vi "Day 2.vi"() -> ()   [LabVIEW 2020]
uses:
  Direction_ENUM.ctl
  a7b40cfa-35c7-42bc-aad7-62f11c57efb3.vi
  <vilib>/Utility/file.llb/Read Delimited Spreadsheet (string).vi
  dc0bc9a9-6357-48e5-90de-08fc84681665.vi
panel:
  out "Position":i32
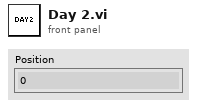
[diagram p1: front panel]
types:
  T1 = typedef "Direction_ENUM.ctl" = enum16{"forward", "up", "down"}
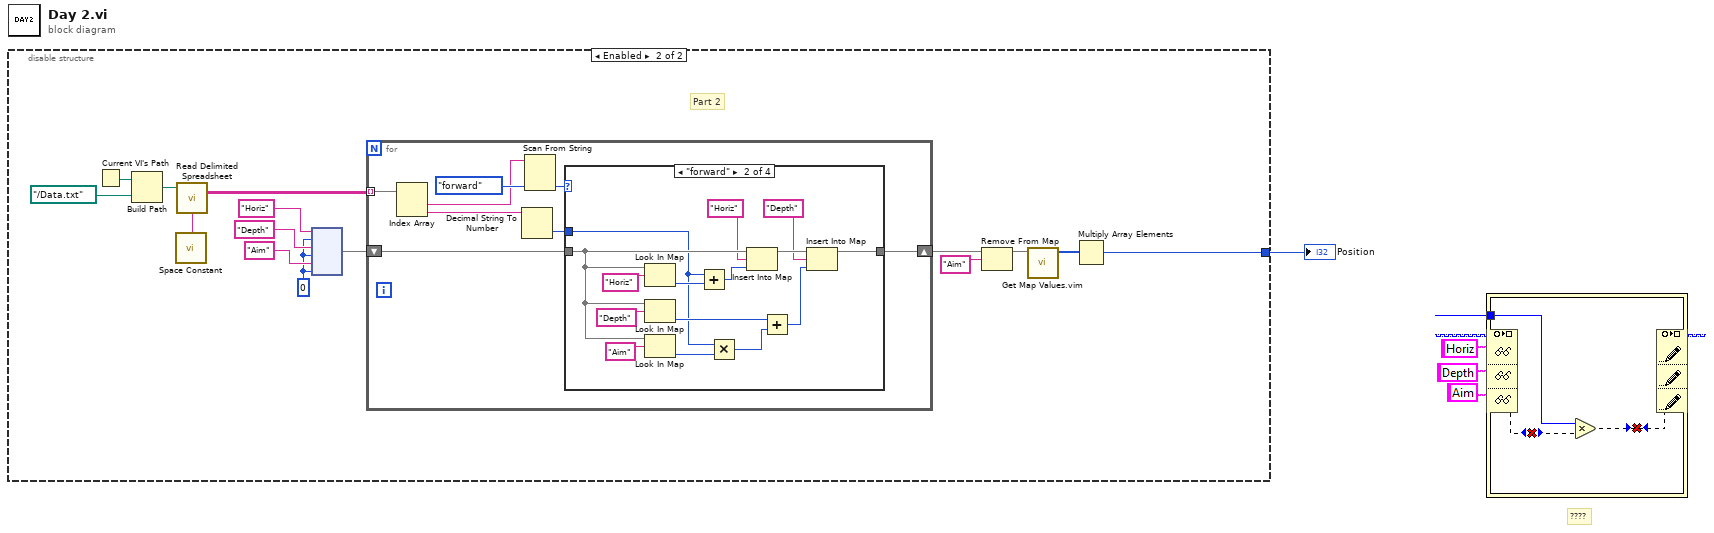
[diagram p0: block diagram]
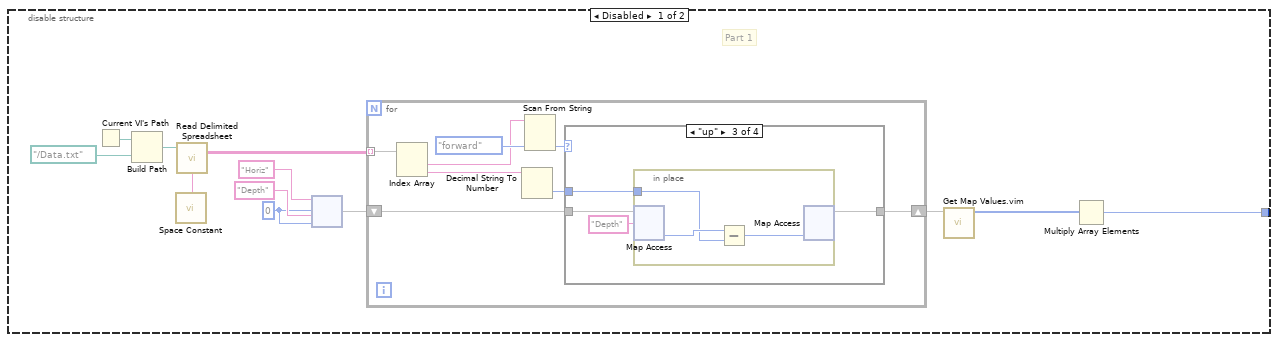
[diagram p2: hidden frame]
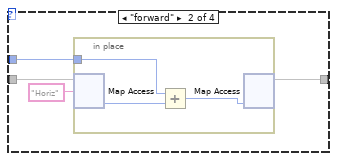
[diagram p4: hidden frame]
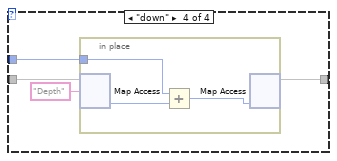
[diagram p5: hidden frame]
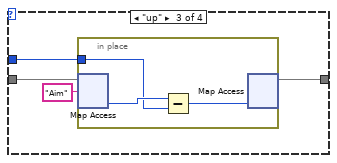
[diagram p7: hidden frame]
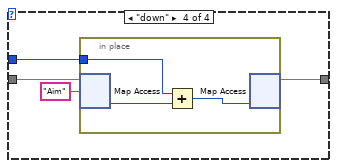
[diagram p8: hidden frame]
diagram:
  # "????"
  n1 = disable-structure shown="Enabled" {
    disable-tunnel: [w2 w44] -> w1
    frame Disabled {
      w6 = 0 ("value")
      # "Part 1"
      n2 = Current VI's Path() -> (path=w12:path)
      n3 = Build Path(base path=w12, name or relative path=path "../Data.txt" ("file path (dialog if empty)")) -> (appended path=w10:path)
      n4 = call <vilib>:"Space Constant.vi"() -> ("String"=w13:string)
      n5 = call-poly <vilib>:"Read Delimited Spreadsheet.vi"("file path (dialog if empty)"=w10, "delimiter (\\t)"=w13) -> ("all rows"=w9:string[][])  [unwired: 8 in, 5 out]
      n6 = node("Horiz" ("key"), w6, "Depth" ("key"), w6) -> (w5:map{string, i32})
      n7 = for {
        tunnel: w9 -> [w21] mode=indexing
        shift-right: [w15] -> w4
        shift-left: w5 -> [w16]
        n8 = Index Array(array=w21) -> (element #1=w18:string, element #2=w20:string)  [unwired: 2 in]
        n9 = Decimal String To Number(string=w20) -> (number=w14:i32)  [unwired: 2 in, 1 out]
        n10 = Scan From String(input string=w18, default 1=Direction_ENUM."forward") -> (output 1=w17:T1)  [unwired: 3 in, 3 out]
        n11 = case shown="\"up\"" w17 {
          tunnel: w16 -> [w22 w26 w31 w38]
          tunnel: [w22 w25 w30 w37] -> w15
          tunnel: w14 -> [_ w24 w32 w39]
          frame Default {
          }
          frame "forward" {
            n12 = in-place {
              in-place-border: w24 -> [w27]
              n13 = in-place-map #1(w26, "Horiz") -> (w29:i32)  [unwired: 1 in, 1 out]
              n14 = Add(x=w27, y=w29) -> (x+y=w28:i32)
              n15 = in-place-map #1(w28) -> (w25:map{string, i32})  [unwired: 1 in, 2 out]
            }
          }
          frame "up" {
            n16 = in-place {
              in-place-border: w32 -> [w34]
              n17 = in-place-map #2(w31, "Depth") -> (w36:i32)  [unwired: 1 in, 1 out]
              n18 = Subtract(x=w36, y=w34) -> (x-y=w35:i32)
              n19 = in-place-map #2(w35) -> (w30:map{string, i32})  [unwired: 1 in, 2 out]
            }
          }
          frame "down" {
            n20 = in-place {
              in-place-border: w39 -> [w41]
              n21 = in-place-map #3(w38, "Depth") -> (w43:i32)  [unwired: 1 in, 1 out]
              n22 = Add(x=w41, y=w43) -> (x+y=w42:i32)
              n23 = in-place-map #3(w42) -> (w37:map{string, i32})  [unwired: 1 in, 2 out]
            }
          }
        }
      }
      n24 = call "Get Map Values.vim"("Map"=w4) -> ("Value Array"=w3:i32[])  [unwired: 10 in]
      n25 = Multiply Array Elements(1:w3) -> (0:w2:i32)
    }
    frame Enabled {
      w48 = 0 ("value")
      # "Part 2"
      n26 = Current VI's Path() -> (path=w57:path)
      n27 = Build Path(base path=w57, name or relative path=path "../Data.txt" ("file path (dialog if empty)")) -> (appended path=w55:path)
      n28 = call <vilib>:"Space Constant.vi"() -> ("String"=w58:string)
      n29 = call-poly <vilib>:"Read Delimited Spreadsheet.vi"("file path (dialog if empty)"=w55, "delimiter (\\t)"=w58) -> ("all rows"=w54:string[][])  [unwired: 8 in, 5 out]
      n30 = node("Horiz" ("key"), w48, "Depth" ("key"), w48, "Aim" ("key"), w48) -> (w51:map{string, i32})
      n31 = for {
        tunnel: w54 -> [w66] mode=indexing
        shift-right: [w60] -> w47
        shift-left: w51 -> [w61]
        n32 = Index Array(array=w66) -> (element #1=w63:string, element #2=w65:string)  [unwired: 2 in]
        n33 = Decimal String To Number(string=w65) -> (number=w59:i32)  [unwired: 2 in, 1 out]
        n34 = Scan From String(input string=w63, default 1=Direction_ENUM."forward") -> (output 1=w62:T1)  [unwired: 3 in, 3 out]
        n35 = case shown="\"forward\"" w62 {
          tunnel: w61 -> [w67 w77 w84 w91]
          tunnel: [w67 w78 w83 w90] -> w60
          tunnel: w59 -> [_ w71 w85 w92]
          frame Default {
          }
          frame "forward" {
            n36 = Look In Map(map=w77, key="Horiz") -> (value=w76:i32)  [unwired: 1 in, 1 out]
            n37 = Look In Map(map=w77, key="Depth") -> (value=w73:i32)  [unwired: 1 in, 1 out]
            n38 = Look In Map(map=w77, key="Aim") -> (value=w70:i32)  [unwired: 1 in, 1 out]
            n39 = Add(x=w71, y=w76) -> (x+y=w75:i32)
            n40 = Multiply(x=w71, y=w70) -> (x*y=w72:i32)
            n41 = Insert Into Map(map in=w77, key="Horiz", value=w75) -> (map out=w79:map{string, i32})  [unwired: 2 out]
            n42 = Add(x=w73, y=w72) -> (x+y=w69:i32)
            n43 = Insert Into Map(map in=w79, key="Depth", value=w69) -> (map out=w78:map{string, i32})  [unwired: 2 out]
          }
          frame "up" {
            n44 = in-place {
              in-place-border: w85 -> [w87]
              n45 = in-place-map #4(w84, "Aim") -> (w89:i32)  [unwired: 1 in, 1 out]
              n46 = Subtract(x=w89, y=w87) -> (x-y=w88:i32)
              n47 = in-place-map #4(w88) -> (w83:map{string, i32})  [unwired: 1 in, 2 out]
            }
          }
          frame "down" {
            n48 = in-place {
              in-place-border: w92 -> [w94]
              n49 = in-place-map #5(w91, "Aim") -> (w96:i32)  [unwired: 1 in, 1 out]
              n50 = Add(x=w94, y=w96) -> (x+y=w95:i32)
              n51 = in-place-map #5(w95) -> (w90:map{string, i32})  [unwired: 1 in, 2 out]
            }
          }
        }
      }
      n52 = Remove From Map(10:"Aim" ("key"), 11:w47) -> (3:w46:map{string, i32})  [unwired: 2 out]
      n53 = call "Get Map Values.vim"("Map"=w46) -> ("Value Array"=w50:i32[])  [unwired: 10 in]
      n54 = Multiply Array Elements(1:w50) -> (0:w44:i32)
    }
  }
  "Position" <- w1
